vi "TwTpsGetNbrModules.vi"(0 "error in (no error)":errorcluster) -> (1 "error out":errorcluster, 2 "nbrModules":i32)   [LabVIEW 2009]
uses:
  Release_Build/TofDaqDll.dll
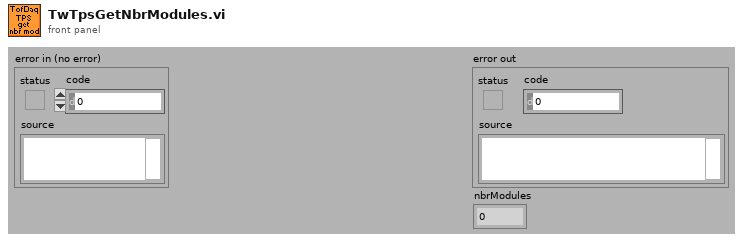
[diagram p1: front panel]
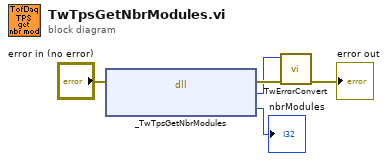
[diagram p0: block diagram]
diagram:
  n1 = dll-call lib="C:/src/TofDaq/Release_Build/TofDaqDll.dll" fn="_TwTpsGetNbrModules"(error in="error in (no error)") -> (error out=w4:errorcluster, "TwRetVal"=w2:i32, "nbrModules"=→"nbrModules":i32)  [unwired: 2 in, 2 out]
  n2 = call "TwErrorConvert.vi"("error in (no error)"=w4, "error code"=w2) -> ("error out"=→"error out":errorcluster)  [unwired: 9 out]
